vi "MultiColumnListbox.vi"(1 "Multicolumn Listbox In":i32(listbox)) -> (0 "Multicolumn Listbox Out":i32(listbox))   [LabVIEW 2010]
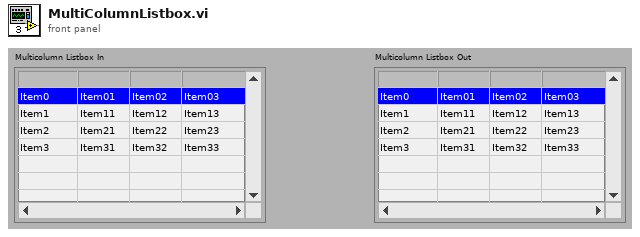
[diagram p1: front panel]
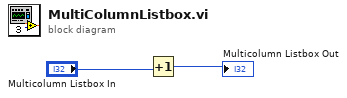
[diagram p0: block diagram]
diagram:
  n1 = Increment(x="Multicolumn Listbox In") -> (x+1=→"Multicolumn Listbox Out":i32)
